vi "Convert Global Decay Fit Parameter Constraints.vi"(8 "Error In":errorcluster, 9 "# Plots":i32, 10 "Fit Model":T1, 11 "Fit Parameter Constraints":T2[](array[typedef]) {"Max Value" format="%#.3g"; "Min Value" format="%#.3g"}) -> (0 "Error Out":errorcluster, 1 "Global Parameters?":bool[](array[boolean]), 3 "Parameter Bounds":T4)   [LabVIEW 2021]
uses:
  AlliGator Decay Fit Parameter Constraints 2.ctl
  Fits/IRF(X)PSED/Decay Fit Parameters In List.ctl
  Fits/Decay Convolution/Decay Model.ctl
  Fits/Fits.lvlib
  AlliGator Decay Fit.lvlib
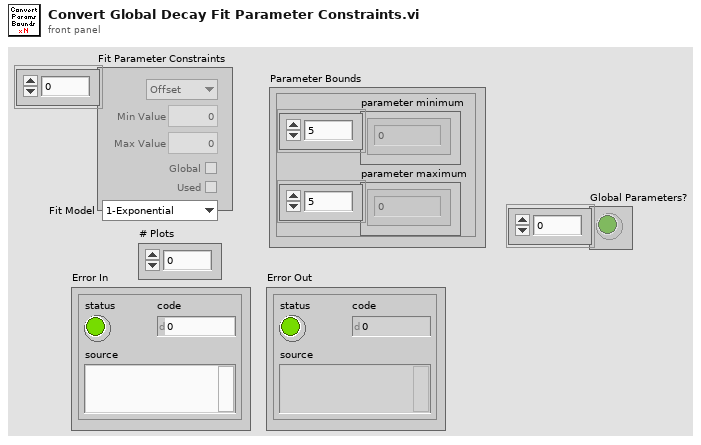
[diagram p1: front panel]
types:
  T1 = typedef "Fits.lvlib/Decay Model.ctl" = enum16{"1-Exponential", "2-Exponentials"}
  T2 = typedef "AlliGator Decay Analysis.lvlib/AlliGator Decay Fit.lvlib/AlliGator Decay Fit Parameter Constraints 2.ctl" = cluster{"Fit Parameter":T3, "Min Value":dbl, "Max Value":dbl, "Global":bool, "Used":bool}
  T3 = typedef "Fits.lvlib/Decay Fit Parameters In List.ctl" = enum16{"Offset", "Baseline", "A_1", "tau_1", "A_2", "tau_2"}
  T4 = cluster{"parameter minimum":dbl[], "parameter maximum":dbl[]}
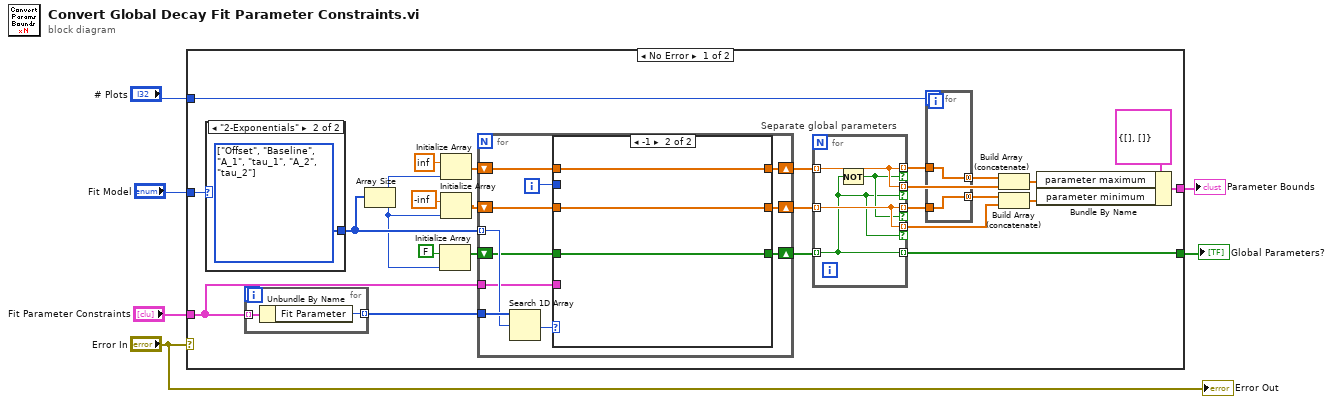
[diagram p0: block diagram]
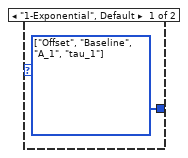
[diagram p2: hidden frame]
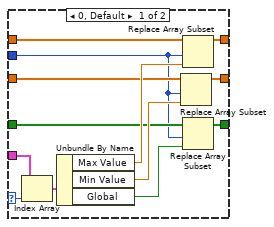
[diagram p3: hidden frame]
diagram:
  n1 = case shown="No Error" "Error In" {
    tunnel: "Fit Parameter Constraints" -> [w26 _]
    tunnel: [w24 _] -> w5
    tunnel: "Fit Model" -> [w23 _]
    tunnel: [w16 _] -> w2
    tunnel: "# Plots" -> [w15 _]
    frame No Error {
      n2 = case shown="\"2-Exponentials\"" w23 {
        tunnel: [w39 w40] -> w31
        frame "1-Exponential", Default {
          w39 = T3[] [enum."Offset", enum."Baseline", enum."A_1", enum."tau_1"] items=["Offset", "Baseline", "A_1", "tau_1", "A_2", "tau_2"] ("Array")
        }
        frame "2-Exponentials" {
          w40 = T3[] [enum."Offset", enum."Baseline", enum."A_1", enum."tau_1", enum."A_2", enum."tau_2"] items=["Offset", "Baseline", "A_1", "tau_1", "A_2", "tau_2"] ("Array")
        }
      }
      n3 = for {
        tunnel: w26 -> [w69] mode=indexing
        tunnel: [w68] -> w32 mode=indexing
        n4 = Unbundle By Name(w69) -> ("Fit Parameter"=w68:T3)
      }
      n5 = Array Size(array=w31) -> (size(s)=w22:i32)
      n6 = Initialize Array(FALSE ("Global"), w22) -> (w20:bool[])
      n7 = Initialize Array(inf ("element"), w22) -> (w29:dbl[])
      n8 = Initialize Array(-inf ("element"), w22) -> (w27:dbl[])
      n9 = for {
        tunnel: w31 -> [w50] mode=indexing
        tunnel: w32 -> [w51]
        shift-right: [w47] -> w19
        shift-left: w29 -> [w48]
        shift-right: [w45] -> w18
        shift-left: w27 -> [w46]
        tunnel: w26 -> [w44]
        shift-right: [w41] -> w17
        shift-left: w20 -> [w42]
        i -> [w43]
        n10 = Search 1D Array(1D array=w51, element=w50) -> (index of element=w49:i32)  [unwired: 1 in]
        n11 = case shown="-1" w49 {
          selector: w49 -> [w64 _]
          tunnel: w48 -> [w61 w67]
          tunnel: [w56 w67] -> w47
          tunnel: w46 -> [w59 w66]
          tunnel: [w57 w66] -> w45
          tunnel: w44 -> [w63 _]
          tunnel: w43 -> [w53 _]
          tunnel: [w54 w65] -> w41
          tunnel: w42 -> [w55 w65]
          frame 0, Default {
            n12 = Index Array(array=w63, index=w64) -> (element=w62:T2)
            n13 = Unbundle By Name(w62) -> ("Max Value"=w60:dbl, "Min Value"=w58:dbl, "Global"=w52:bool)
            n14 = Replace Array Subset(array=w59, new element=w58, index=w53) -> (w57:dbl[])
            n15 = Replace Array Subset(array=w61, new element=w60, index=w53) -> (w56:dbl[])
            n16 = Replace Array Subset(array=w55, new element=w52, index=w53) -> (w54:bool[])
          }
          frame -1 {
          }
        }
      }
      n17 = for "Separate global parameters" {
        tunnel: w19 -> [w37] mode=indexing
        tunnel: w18 -> [w38] mode=indexing
        tunnel: w17 -> [w35] mode=indexing
        tunnel: [w37] -> w14 mode=indexing if=w36
        tunnel: [w38] -> w13 mode=indexing if=w36
        tunnel: [w35] -> w16 mode=indexing
        tunnel: [w38] -> w7 mode=indexing if=w35
        tunnel: [w37] -> w8 mode=indexing if=w35
        n18 = Not(x=w35) -> (.not. x?=w36:bool)
      }
      n19 = for {
        N: w15 -> [_]
        tunnel: w14 -> [w34]
        tunnel: w13 -> [w33]
        tunnel: [w34] -> w12 mode=concatenating
        tunnel: [w33] -> w11 mode=concatenating
      }
      n20 = Build Array (concatenate)(w12, w8) -> (w10:dbl[])
      n21 = Build Array (concatenate)(w11, w7) -> (w9:dbl[])
      n22 = Bundle By Name(cluster=T4 {"parameter minimum"=[], "parameter maximum"=[]} ("parameter bounds"), "parameter maximum"=w10, "parameter minimum"=w9) -> (w24:T4)
    }
    frame Error {
    }
  }
  "Parameter Bounds" <- w5
  "Global Parameters?" <- w2
  "Error Out" <- "Error In"
